vi "file_path.vi"(8 "error in (no error)":errorcluster) -> (0 "error out":errorcluster, 1 "app file extension":string, 2 "app name":string, 3 "app toml path":path)   [LabVIEW 2017, in "toml.lvlib"]
uses:
  toml.lvlib
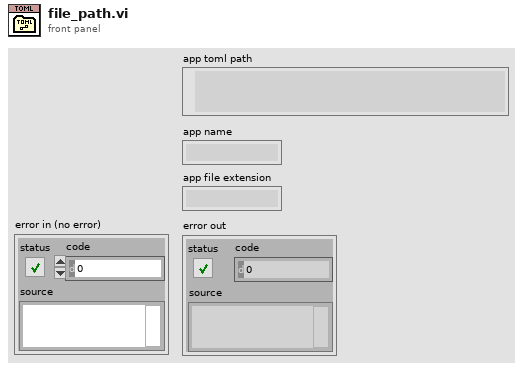
[diagram p1: front panel]
types:
  T1 = enum32{"invalid app kind", "Development System", "Run Time System", "Student Edition", "Embedded LabVIEW", "Evaluation", "Custom"}
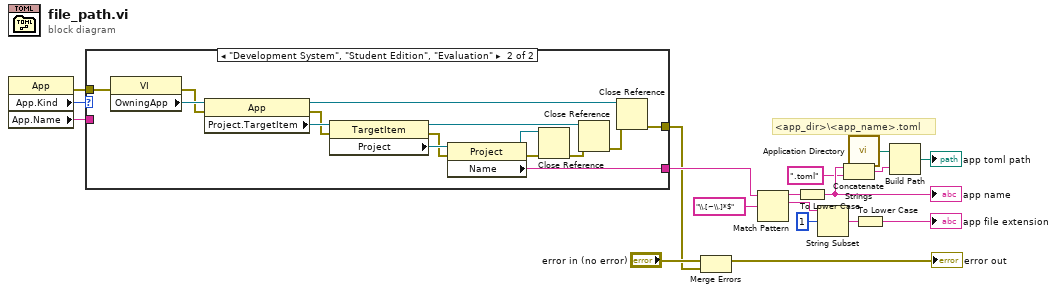
[diagram p0: block diagram]
diagram:
  # "<app_dir>\\<app_name>.toml"
  n1 = property class="App"() -> (error out=w8:errorcluster, "App.Kind"=w11:T1, "App.Name"=w10:string)  [unwired: 2 in, 1 out]
  n2 = case shown="\"Development System\", \"Student Edition\", \"Evaluation\"" w11 {
    tunnel: w10 -> [w20 _]
    tunnel: [w20 w22] -> w9
    tunnel: w8 -> [w19 w35]
    tunnel: [w19 w21] -> w1
    frame "invalid app kind", "Run Time System", "Embedded LabVIEW", "Custom" {
    }
    frame "Development System", "Student Edition", "Evaluation" {
      n3 = property class="VI"(error in=w35) -> (error out=w33:errorcluster, "OwningApp"=w34:refnum<vi>)  [unwired: 1 in, 1 out]
      n4 = property class="App"(reference=w34, error in=w33) -> (reference out=w24:refnum<vi>, error out=w31:errorcluster, "Project.TargetItem"=w32:refnum<vi>)
      n5 = property class="TargetItem"(reference=w32, error in=w31) -> (reference out=w26:refnum<vi>, error out=w29:errorcluster, "Project"=w30:refnum<vi>)
      n6 = property class="Project"(reference=w30, error in=w29) -> (reference out=w27:refnum<vi>, error out=w28:errorcluster, "Name"=w22:string)
      n7 = Close Reference(reference=w27, error in (no error)=w28) -> (error out=w25:errorcluster)
      n8 = Close Reference(reference=w26, error in (no error)=w25) -> (error out=w23:errorcluster)
      n9 = Close Reference(reference=w24, error in (no error)=w23) -> (error out=w21:errorcluster)
    }
  }
  n10 = Merge Errors("error in (no error)", w1) -> (→"error out":errorcluster)
  n11 = Match Pattern(string=w9, regular expression="\\.[~\\.]*$") -> (before substring=w14:string, match substring=w7:string)  [unwired: 3 out]
  n12 = To Lower Case(string=w14) -> (all lower case string=w18:string)
  "app name" <- w18
  n13 = String Subset(string=w7, offset (0)=1) -> (substring=w5:string)  [unwired: 1 in]
  n14 = Concatenate Strings(w18, ".toml" ("string")) -> (w15:string)
  n15 = call <vilib>:"Application Directory.vi"() -> ("Application Directory"=w12:path)
  n16 = To Lower Case(string=w5) -> (all lower case string=→"app file extension":string)
  n17 = Build Path(base path=w12, name or relative path=w15) -> (appended path=→"app toml path":path)
